vi "set plugin info.vi"(8 "error in (no error)":errorcluster, 9 "plugin info":T1, 10 "id":string, 11 "DSFConfiguration in":refnum<class "DSFConfiguration.lvclass">) -> (0 "error out":errorcluster, 3 "DSFConfiguration out":refnum<class "DSFConfiguration.lvclass">)   [LabVIEW 2017, in "DSFConfiguration.lvclass"]
uses:
  DSFConfiguration.lvclass
  Controls/dsf configuration file/1.0.0/dsf timing.ctl
  Controls/dsf configuration file/1.0.0/dsf configuration file v1.0.0.lvlib
  Controls/dsf configuration file/1.0.0/dsf plugin.ctl
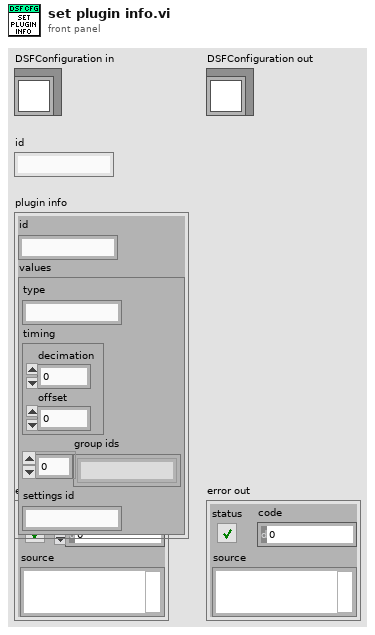
[diagram p1: front panel]
types:
  T1 = typedef "dsf configuration file v1.0.0.lvlib/dsf plugin.ctl" = cluster{"id":string, "values":cluster{"type":string, "timing":T2, "group ids":string[], "settings id":string}}
  T2 = typedef "dsf configuration file v1.0.0.lvlib/dsf timing.ctl" = cluster{"decimation":i32, "offset":i32}
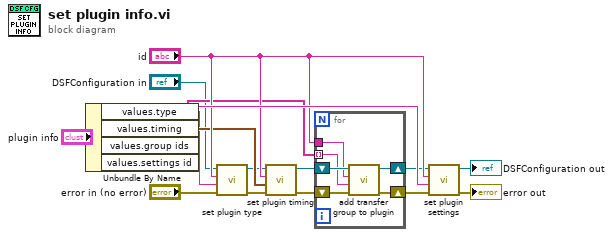
[diagram p0: block diagram]
diagram:
  n1 = Unbundle By Name("plugin info") -> ("values.type"=w5:string, "values.timing"=w8:T2, "values.group ids"=w11:string[], "values.settings id"=w16:string)
  n2 = call "set plugin type.vi"("error in (no error)"="error in (no error)", "plugin type"=w5, "id"="id", "DSFConfiguration in"="DSFConfiguration in") -> ("error out"=w3:errorcluster, "DSFConfiguration out"=w7:refnum<class "DSFConfiguration.lvclass">)  [unwired: 6 in]
  n3 = call "set plugin timing.vi"("error in (no error)"=w3, "timing info"=w8, "id"="id", "DSFConfiguration in"=w7) -> ("error out"=w6:errorcluster, "DSFConfiguration out"=w10:refnum<class "DSFConfiguration.lvclass">)  [unwired: 6 in]
  n4 = for {
    tunnel: "id" -> [w18]
    tunnel: w11 -> [w17] mode=indexing
    shift-right: [w21] -> w9
    shift-left: w6 -> [w22]
    shift-right: [w19] -> w13
    shift-left: w10 -> [w20]
    n5 = call "add transfer group to plugin.vi"("error in (no error)"=w22, "transfer group id"=w17, "id"=w18, "DSFConfiguration in"=w20) -> ("error out"=w21:errorcluster, "DSFConfiguration out"=w19:refnum<class "DSFConfiguration.lvclass">)  [unwired: 6 in]
  }
  n6 = call "set plugin settings.vi"("error in (no error)"=w9, "settings id"=w16, "id"="id", "DSFConfiguration in"=w13) -> ("error out"=→"error out":errorcluster, "DSFConfiguration out"=→"DSFConfiguration out":refnum<class "DSFConfiguration.lvclass">)  [unwired: 6 in]
